vi "Read output.vi"(8 "error in (no error)":errorcluster, 11 "IOCard in":refnum<class "IOCard.lvclass">) -> (0 "error out":errorcluster, 2 "output":bool[](array[boolean]), 3 "IOCard out":refnum<class "IOCard.lvclass">)   [LabVIEW 2019, in "IOCard.lvclass"]
uses:
  IOCard.lvclass
  IOCard.lvclass/IOCard.ctl
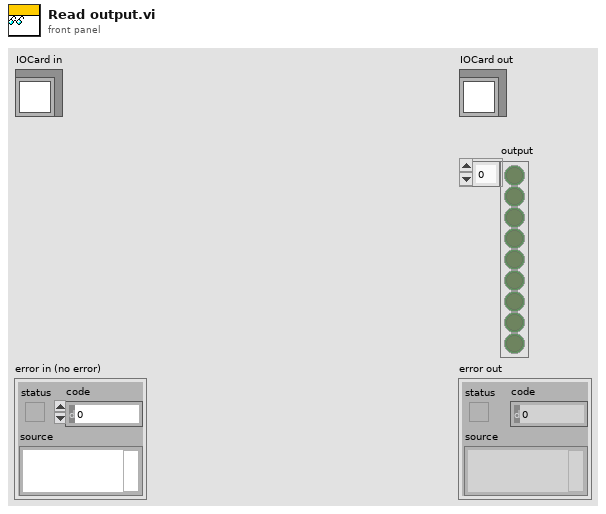
[diagram p1: front panel]
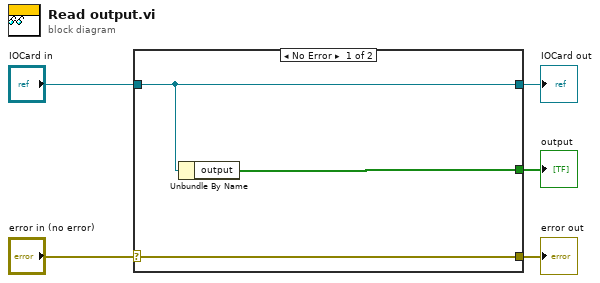
[diagram p0: block diagram]
diagram:
  n1 = case shown="No Error" "error in (no error)" {
    selector: "error in (no error)" -> [w8 w9]
    tunnel: [w8 w9] -> w4
    tunnel: [w7 w10] -> w2
    tunnel: "IOCard in" -> [w7 w10]
    tunnel: [w6 _] -> w1
    frame No Error {
      n2 = Unbundle By Name(w7) -> ("output"=w6:bool[])
    }
    frame Error {
    }
  }
  "error out" <- w4
  "IOCard out" <- w2
  "output" <- w1
